vi "Find TSC tEXt Chunk.vi"(6 "Save if not found?":bool, 8 "error in":errorcluster, 10 "file path (use dialog)":path) -> (0 "error out":errorcluster, 1 "Found?":bool, 2 "file path dup":path)   [LabVIEW 2026, in "TSC Material Theme.lvlib" / "Material-Scheme.lvclass"]
doc: "Look to see if the TSC author tag has been embedded into the PNG\n\n<b>Code Developed By:</b> +\nDaniel Coons +\nTechnology Service Corporation +\nwww.tsc.com/atcs"
uses:
  Material-Scheme.lvclass
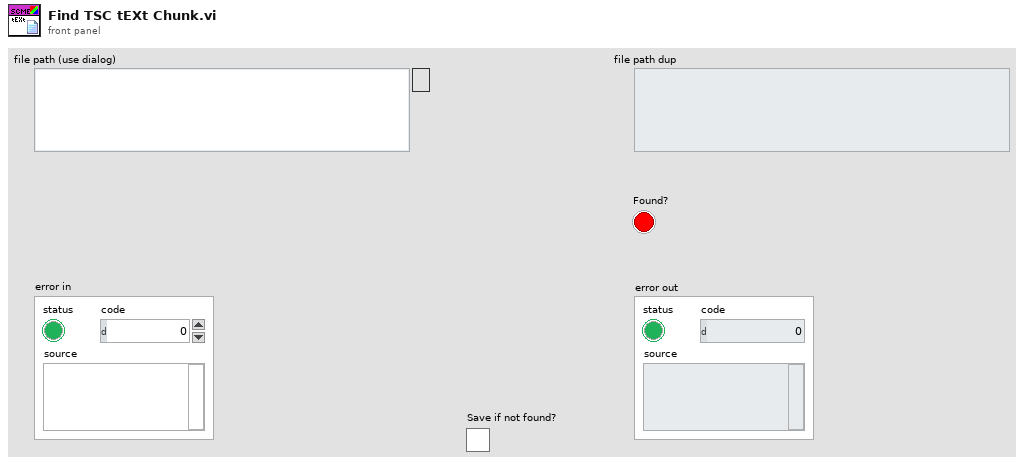
[diagram p1: front panel]
types:
  T1 = enum16{"open", "replace", "create", "open or create", "replace or create", "replace or create with confirmation"}
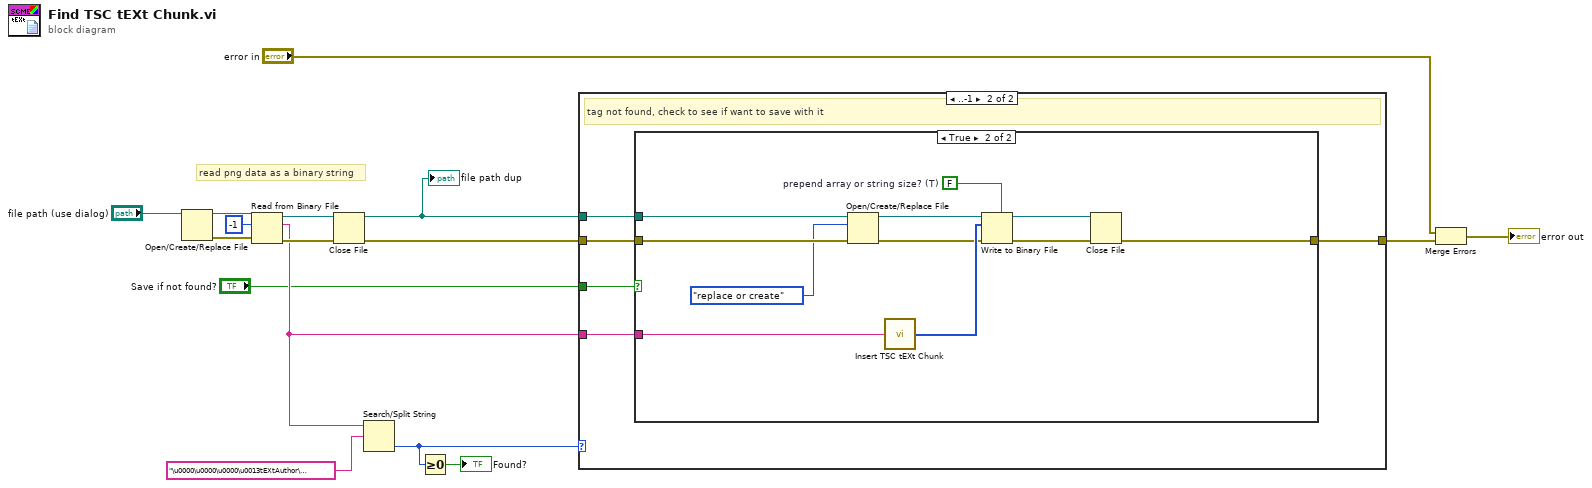
[diagram p0: block diagram]
diagram:
  # "read png data as a binary string"
  n1 = Open/Create/Replace File(file path (use dialog)="file path (use dialog)") -> (refnum out=w16:refnum<file>, error out=w15:errorcluster)  [unwired: 5 in, 1 out]
  n2 = Read from Binary File(8:w15, 10:-1 ("count (1)"), 11:w16) -> (0:w13:errorcluster, 2:w9:string, 3:w14:refnum<file>)  [unwired: 3 in, 1 out]
  n3 = Close File(refnum=w14, error in=w13) -> (path=w1:path, error out=w11:errorcluster)
  "file path dup" <- w1
  n4 = Search/Split String(string=w9, search string/char (-)="\u0000\u0000\u0000\u0013tEXtAuthor\u0000tscicondecal^Ø" ("string")) -> (offset of match=w5:i32)  [unwired: 1 in, 2 out]
  n5 = Greater Or Equal To 0?(x=w5) -> (x >= 0?=→"Found?":bool)
  n6 = case shown="..-1" w5 {
    tunnel: w11 -> [w17 w22]
    tunnel: w9 -> [_ w21]
    tunnel: [w17 w20] -> w7
    tunnel: "Save if not found?" -> [_ w19]
    tunnel: w1 -> [_ w18]
    frame Default {
      # "found, do nothing"
    }
    frame ..-1 {
      # "tag not found, check to see if want to save with it"
      n7 = case shown="True" w19 {
        tunnel: w22 -> [w23 w34]
        tunnel: w21 -> [_ w33]
        tunnel: [w23 w32] -> w20
        tunnel: w18 -> [_ w24]
        frame False {
        }
        frame True {
          w25 = FALSE  # prepend array or string size? (T)
          n8 = Open/Create/Replace File(file path (use dialog)=w24, error in=w34, operation (0:open)=T1."replace or create") -> (refnum out=w27:refnum<file>, error out=w28:errorcluster)  [unwired: 3 in, 1 out]
          n9 = call "Insert TSC tEXt Chunk.vi"("png binary string"=w33) -> ("New PNG Binary"=w31:u8[])
          n10 = Write to Binary File(file (use dialog)=w27, data=w31, error in=w28, 5:w25) -> (refnum out=w29:refnum<file>, error out=w26:errorcluster)  [unwired: 2 in, 1 out]
          n11 = Close File(refnum=w29, error in=w26) -> (error out=w32:errorcluster)  [unwired: 1 out]
        }
      }
    }
  }
  n12 = Merge Errors("error in", w7) -> (→"error out":errorcluster)
